vi "_Create (Protected).vi"(8 "error in (no error)":errorcluster, 11 "ListImp in":refnum<class "ListImp.lvclass">) -> (0 "error out":errorcluster, 3 "ListImp out":refnum<class "ListImp.lvclass">)   [LabVIEW 2017, in "LapDog.Collections.v0.Lists.lvlib" / "ListImp.lvclass"]
doc: "This method is invoked when the List:Create method is called. Child implementations should override this method to initialize or obtain any runtime resource needed."
uses:
  ListImp.lvclass
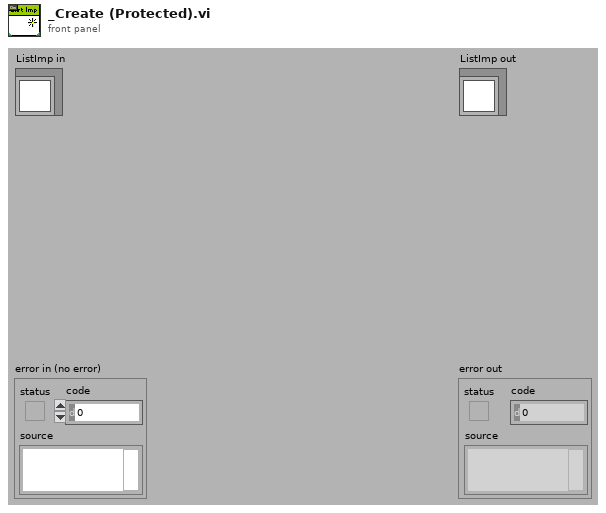
[diagram p1: front panel]
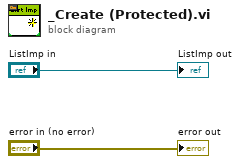
[diagram p0: block diagram]
diagram:
  "error out" <- "error in (no error)"
  "ListImp out" <- "ListImp in"
